vi "Cholesky Factorization Rank-1 Update_Update (DBL).vi"(10 "X":dbl[](array[numeric]), 11 "R":T1) -> (3 "Updated R":T1)   [LabVIEW 2020, in "NI_AAL_LinAlg.lvlib"]
uses:
  <vilib>/Analysis/NI_AAL_LinAlg.lvlib
  <vilib>/Analysis/Matrix/Datatypes/RealMatrix.ctl
  <vilib>/Analysis/Matrix/NI_Matrix.lvlib
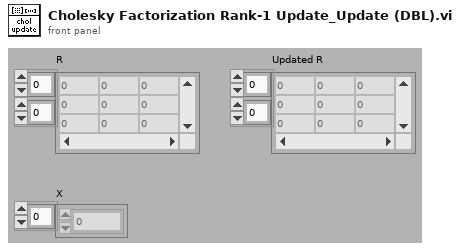
[diagram p1: front panel]
types:
  T1 = typedef "NI_Matrix.lvlib/RealMatrix.ctl" = dbl[][]
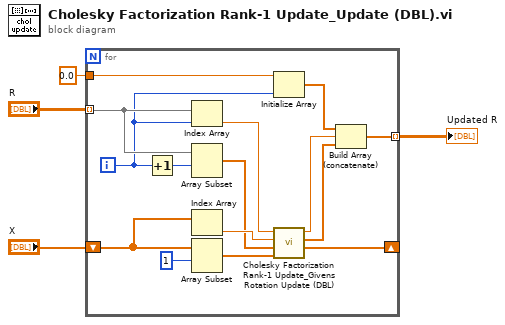
[diagram p0: block diagram]
diagram:
  n1 = for {
    shift-right: [w5] -> _
    shift-left: "X" -> [w18]
    tunnel: "R" -> [w17] mode=indexing
    tunnel: [w14] -> w1 mode=indexing
    tunnel: 0.0 -> [w7]
    i -> [w13]
    n2 = Increment(x=w13) -> (x+1=w16:i32)
    n3 = Index Array(array=w17, index=w13) -> (element=w12:dbl)
    n4 = Array Subset(array=w17, index=w16) -> (w9:dbl[])  [unwired: 1 in]
    n5 = Index Array(array=w18) -> (element=w11:dbl)  [unwired: 1 in]
    n6 = Array Subset(array=w18, index=1) -> (w10:dbl[])  [unwired: 1 in]
    n7 = Initialize Array(w7, w13) -> (w19:dbl[])
    n8 = call <vilib>:"Cholesky Factorization Rank-1 Update_Givens Rotation Update (DBL).vi"("Y In"=w10, "X In"=w9, "b"=w11, "a"=w12) -> ("Y Out"=w5:dbl[], "X Out"=w6:dbl[], "v"=w8:dbl)  [unwired: 5 in]
    n9 = Build Array (concatenate)(w19, w8, w6) -> (w14:dbl[])
  }
  "Updated R" <- w1
